vi "Full Autonmous Scripted V1.vi"(8 "error in":errorcluster) -> ()   [LabVIEW 2013]
uses:
  Robot Global Var.vi
  Auto text File Code/Autonmous Scripting array typedef.ctl
  Auto text File Code/Autonmous Program typedef.ctl
  Auto text File Code/All Autonmous Programs typedef.ctl
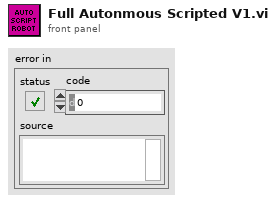
[diagram p1: front panel]
types:
  T1 = typedef "All Autonmous Programs typedef.ctl" = cluster{"All Scripting data":T2[], "Auto Names":string[]}
  T2 = typedef "Autonmous Program typedef.ctl" = cluster{"Autonmous name":string, "Auto Scripting array":T3}
  T3 = typedef "Autonmous Scripting array typedef.ctl" = string[]
  T4 = typedef "Robot dev revs.ctl" = cluster{"Drive":T5, "Roller dev revs":cluster{"Roller devs":cluster{"SolenoidDevRef":T15, "MotorControlDeviceRef":T8}}, "Catapult devrevs":T26, "CompressorDevRef":T29, "Drive Joystick":T33, "Operator Joystick":T33}
  T5 = typedef "Drive typedef.ctl" = cluster{"Drive Actuaters":cluster{"Motor devRevs":T6, "SolenoidDevRef":T15}, "Drive Sensor data":T18}
  T6 = typedef "Drive Motors Typedef.ctl" = cluster{"Left Side Motors":T7, "Right Side Motors":T7, "dev Status":errorcluster}
  T7 = typedef "GearBox Typedef.ctl" = cluster{"Motor 1 devRev":T8, "Motor 2 devRev":T8, "Motor 3 devRev":T8}
  T8 = typedef "WPI_MotorControlDeviceRef.ctl" = cluster{"DeviceStatus":errorcluster, "Type":enum16{"PWM", "CAN"}, "PWM":cluster{"Digital Module":T9, "PWM Channel":T10, "DeadBand":T11}, "CAN":cluster{"Device Number":u8, "Control Mode":T12, "Semaphore":T13, "Max Vout":dbl}, "Invert":bool, "TransformRef":T14, "InvTransformRef":T14}
  T9 = typedef "FPGA_TypedefDigitalModule.ctl" = enum16{"Digital Module 1", "Digital Module 2"}
  T10 = typedef "FPGA_DIOPWMChannel.ctl" = enum8{"PWM 1", "PWM 2", "PWM 3", "PWM 4", "PWM 5", "PWM 6", "PWM 7", "PWM 8", "PWM 9", "PWM 10", "Invalid"}
  T11 = typedef "WPI_PWMDeadband.ctl" = cluster{"Name":string, "maxPositivePwm":i32, "minPositivePwm":i32, "centerPwm":i32, "maxNegativePwm":i32, "minNegativePwm":i32, "angularRange":u16}
  T12 = typedef "WPI_CANJaguar_ControlMode.ctl" = enum8{"Percent VBus", "Current", "Speed", "Position", "Voltage"}
  T13 = typedef "Semaphore RefNum" = refnum<k1>
  T14 = typedef "WPI_PWMTransform_ConPane.ctl" = refnum<vi>
  T15 = typedef "WPI_SolenoidDevRef.ctl" = cluster{"DevStatus":errorcluster, "Solenoid Module":T16, "Forward Solenoid Channel":T17, "Reverse Solenoid Channel":T17}
  T16 = typedef "FPGA_TypedefSolenoidModule.ctl" = enum16{"Solenoid Module 1", "Solenoid Module 2"}
  T17 = typedef "WPI_SolenoidChannel.ctl" = enum8{"Solenoid 1", "Solenoid 2", "Solenoid 3", "Solenoid 4", "Solenoid 5", "Solenoid 6", "Solenoid 7", "Solenoid 8", "Invalid"}
  T18 = typedef "Drive Sensor Typedef.ctl" = cluster{"Encoders":cluster{"Left Encoder":T19, "Right Encoder":T19}, "GyroDevRef":T23, "Last commanded Angle":dbl}
  T19 = typedef "WPI_EncoderDevRef.ctl" = cluster{"DevStatus":errorcluster, "EncoderIndex":T20, "CounterIndex":T21, "DistancePerCount":dbl, "Decoding Type":T22}
  T20 = typedef "FPGA_EncoderIdx.ctl" = enum8{"Enc 0", "Enc 1", "Enc 2", "Enc 3", "Invalid"}
  T21 = typedef "FPGA_CounterCtrSystemIndex.ctl" = enum8{"Ctr 0", "Ctr 1", "Ctr 2", "Ctr 3", "Ctr 4", "Ctr 5", "Ctr 6", "Ctr 7", "Invalid"}
  T22 = typedef "WPI_EncoderType.ctl" = enum16{"1x", "2x", "4x"}
  T23 = typedef "WPI_GyroDevRef.ctl" = cluster{"DevStatus":errorcluster, "Analog Module":T24, "Analog Channel":T25, "Offset":dbl, "Gain (VoltsPerDegree/Second)":dbl}
  T24 = typedef "FPGA_TypedefAnalogModule.ctl" = enum16{"Analog Module 1", "Analog Module 2"}
  T25 = typedef "FPGA_AIChannel.ctl" = enum8{"AI 1", "AI 2", "AI 3", "AI 4", "AI 5", "AI 6", "AI 7", "AI 8", "Invalid"}
  T26 = typedef "catapult type def.ctl" = cluster{"MotorControlDeviceRef":T8, "SolenoidDevRef":T15, "DigitalInputDevRef":T27}
  T27 = typedef "WPI_DigitalInputDevRef.ctl" = cluster{"DevStatus":errorcluster, "DIO Channel":T28, "Digital Module":T9}
  T28 = typedef "FPGA_DIOChannel.ctl" = enum8{"DIO 1", "DIO 2", "DIO 3", "DIO 4", "DIO 5", "DIO 6", "DIO 7", "DIO 8", "DIO 9", "DIO 10", "DIO 11", "DIO 12", "DIO 13", "DIO 14", "Invalid"}
  T29 = typedef "WPI_CompressorDevRef.ctl" = cluster{"DevStatus":errorcluster, "DigitalInputDevRef":T27, "RelayDevRef":T30}
  T30 = typedef "WPI_RelayDevRef.ctl" = cluster{"DevStatus":errorcluster, "Relay Channel":T31, "Digital Module":T9, "Relay Direction":T32}
  T31 = typedef "FPGA_DIORelayChannel.ctl" = enum8{"Relay 1", "Relay 2", "Relay 3", "Relay 4", "Relay 5", "Relay 6", "Relay 7", "Relay 8", "Invalid"}
  T32 = typedef "WPI_RelayDirection.ctl" = enum16{"Both directions", "Forward only", "Reverse only"}
  T33 = typedef "WPI_JoystickDevRef.ctl" = cluster{"Device":T34}
  T34 = typedef "WPI_JoystickDeviceEnum.ctl" = enum16{"USB 1", "USB 2", "USB 3", "USB 4", "Kinect 1", "Kinect 2"}
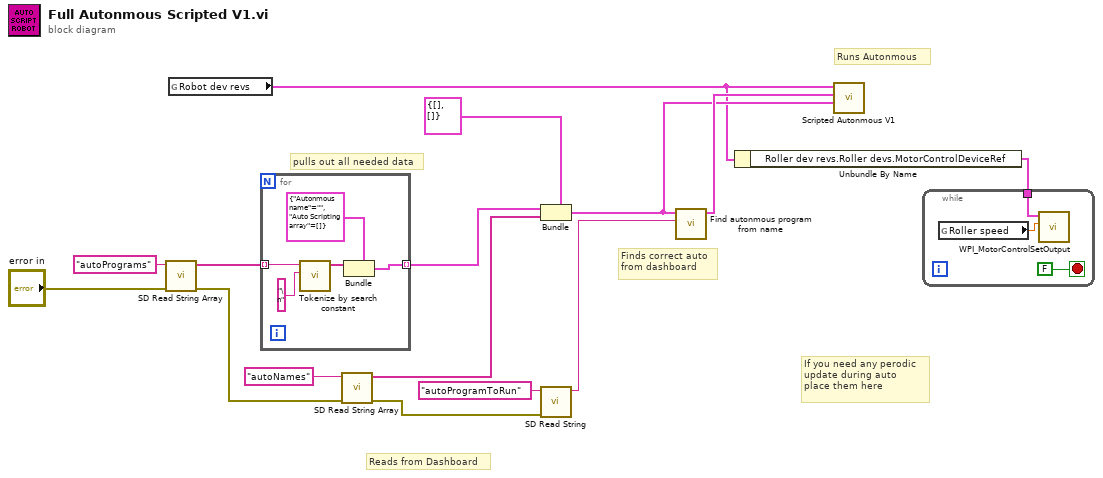
[diagram p0: block diagram]
diagram:
  # "If you need any perodic\nupdate during auto\nplace them here"
  # "Runs Autonmous"
  # "pulls out all needed data"
  # "Finds correct auto\nfrom dashboard"
  # "Reads from Dashboard"
  n1 = call <vilib>:"SD Read String Array.vi"("error in"="error in", "Name"="autoPrograms") -> ("error out"=w7:errorcluster, "String Array"=w12:string[])  [unwired: 8 in]
  n2 = global read "Robot Global Var.vi" "Robot dev revs"() -> (w2:T4)
  n3 = for {
    tunnel: w12 -> [w19] mode=indexing
    tunnel: [w17] -> w10 mode=indexing
    n4 = call "Tokenize by search constant.vi"("search constant"="\n", "Data"=w19) -> ("Array"=w18:string[])  [unwired: 9 in]
    n5 = Bundle(cluster=T2 {"Autonmous name"="", "Auto Scripting array"=[]} ("Autonmous Program"), "Autonmous name"=w18) -> (w17:T2)  [unwired: 1 in]
  }
  n6 = call <vilib>:"SD Read String Array.vi"("error in"=w7, "Name"="autoNames") -> ("error out"=w8:errorcluster, "String Array"=w9:string[])  [unwired: 8 in]
  n7 = Bundle(cluster=T1 {"All Scripting data"=[], "Auto Names"=[]} ("All Autonmous Programs"), "All Scripting data"=w10, "Auto Names"=w9) -> (w3:T1)
  n8 = call <vilib>:"SD Read String.vi"("error in"=w8, "Name"="autoProgramToRun") -> ("String"=w5:string)  [unwired: 7 in, 2 out]
  n9 = call "Find autonmous program from name.vi"("Program Name"=w5, "All Autonmous Programs"=w3) -> ("Autonmous Program"=w4:T2)  [unwired: 8 in, 1 out]
  n10 = Unbundle By Name(w2) -> ("Roller dev revs.Roller devs.MotorControlDeviceRef"=w1:T8)
  n11 = call "Scripted Autonmous V1.vi"("All Autonmous Programs"=w3, "Autonmous Program"=w4, "Robot dev revs"=w2) -> ()  [unwired: 8 in, 1 out]
  n12 = while {
    tunnel: w1 -> [w23]
    stop <- FALSE stop-if-true
    n13 = global read "Robot Global Var.vi" "Roller speed"() -> (w22:dbl)
    n14 = call <vilib>:"WPI_MotorControlSetOutput.vi"("Output"=w22, "MotorControlDevRef"=w23) -> ()  [unwired: 7 in, 3 out]
  }
